vi "Read or Write Bookmark (XML file).vi"(1 "Read or write":enum16{"Read", "Write"}(ring)=enum."Write", 2 "Type":T1, 5 "PDF path file":path=path "C:/Users/JMS/Documents/PDF Report/Essais pdf/User Manual.pdf", 7 "XML File":path=path "C:/Users/JMS/Documents/PDF Report/Essais pdf/outline_actions31.xml", 11 "error in (no error)":errorcluster) -> (4 "GetBookmark":refnum<k24>, 6 "Bookmark?":bool, 8 "XML File duplicate":path=path "C:/Users/JMS/Documents/PDF Report/Essais pdf/outline_actions31.xml", 15 "error out":errorcluster)   [LabVIEW 2019, in "Exaprom PDF.lvlib"]
doc: "Version 1.1\nDeveloped by Jean-Marc Simard\nCopyright © 2012, Exaprom Inc.\nAll rights reserved.\nLicense: BSD\n\nWith iTextSharp 4.1.6 (http://itextsharp.sourceforge.net)\nunder Mozilla Public License Version 1.1\n(http://www.mozilla.org/MPL/MPL-1.1.html)"
uses:
  Controls/Text Controls/Unicode/Character type.ctl
  Controls/General Controls/Create, open or close.ctl
  Controls/Concatenate Controls/PDF file to concatenate.ctl
  C:/work/niobrara_lv/labview pdf writer fixing/DLL/itextsharp.dll
  DLL/itextsharp.dll
  Exaprom PDF.lvlib
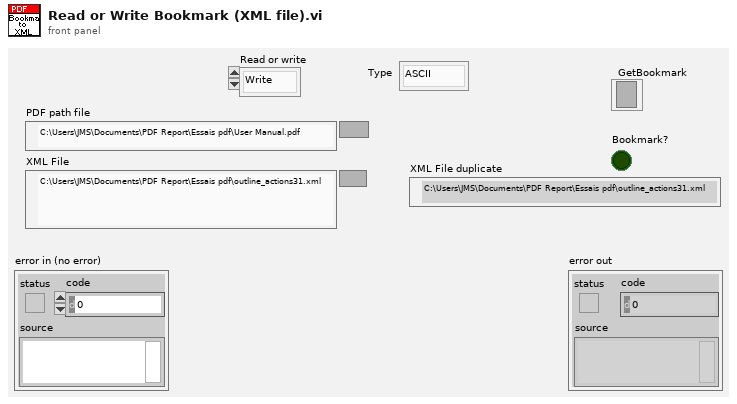
[diagram p1: front panel]
types:
  T1 = typedef "Exaprom PDF.lvlib/Character type.ctl" = enum16{"ASCII", "Unicode"}
  T2 = typedef "Exaprom PDF.lvlib/PDF file to concatenate.ctl" = cluster{"Path":path, "Pages":string, "Password":string}
  T3 = typedef "Exaprom PDF.lvlib/Create, open or close.ctl" = enum16{"Create", "Open", "Close"}
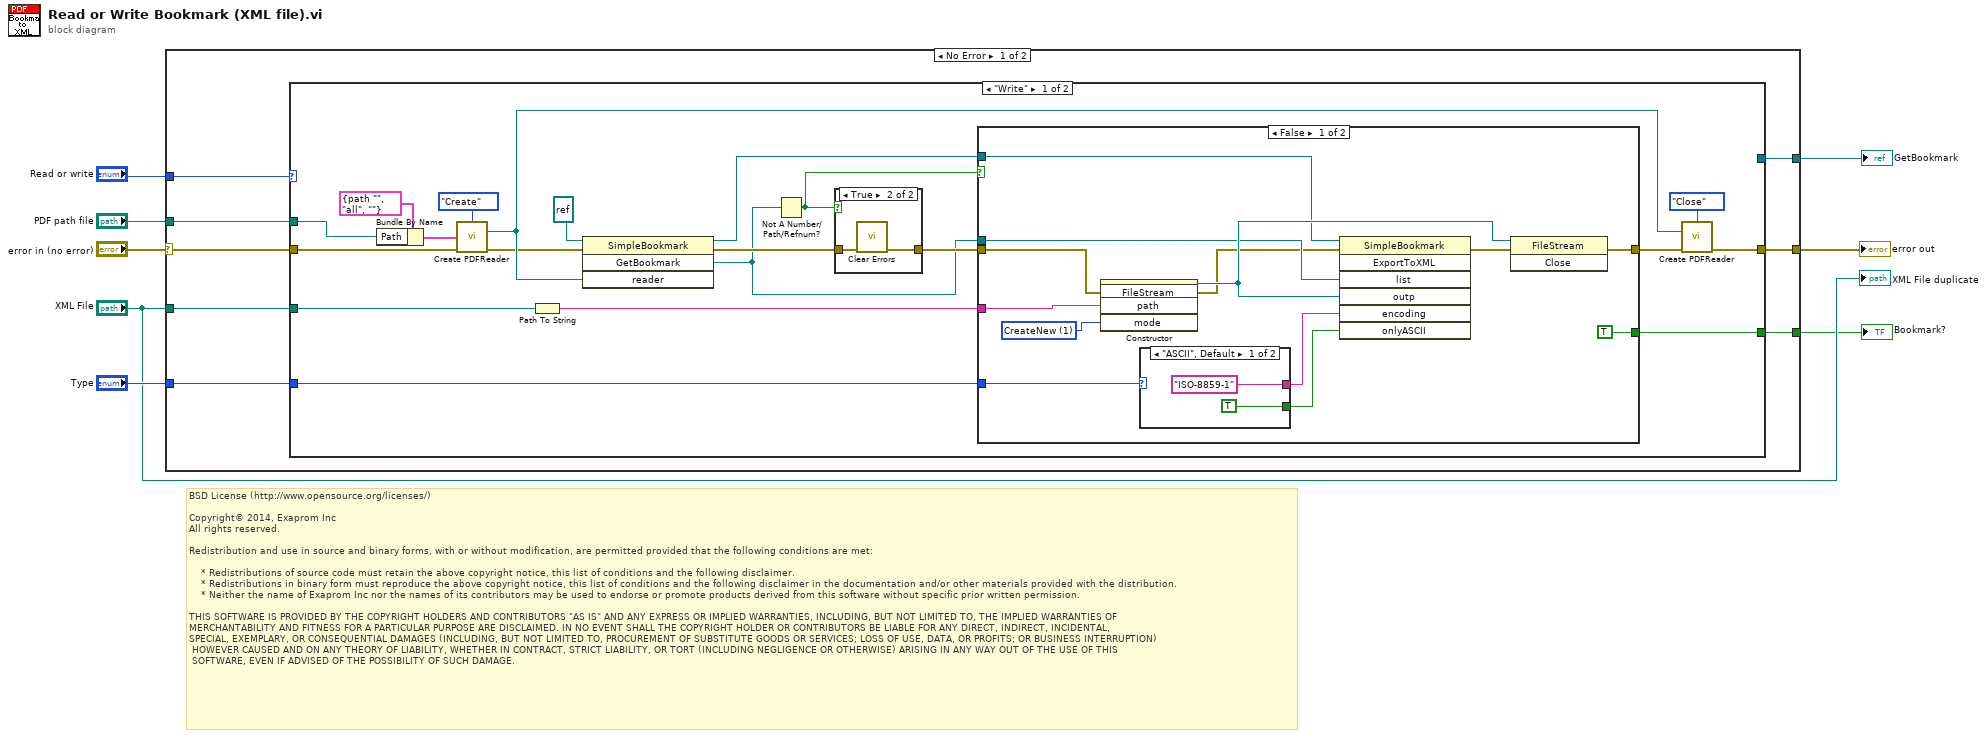
[diagram p0: block diagram]
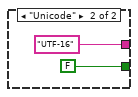
[diagram p3: hidden frame]
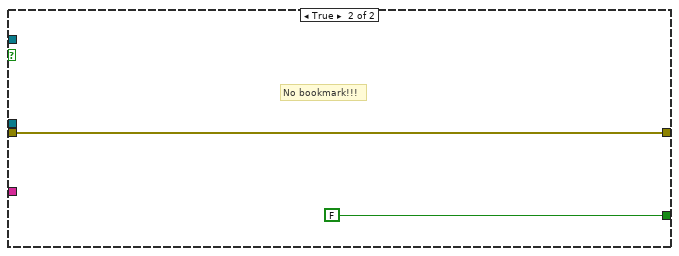
[diagram p4: hidden frame]
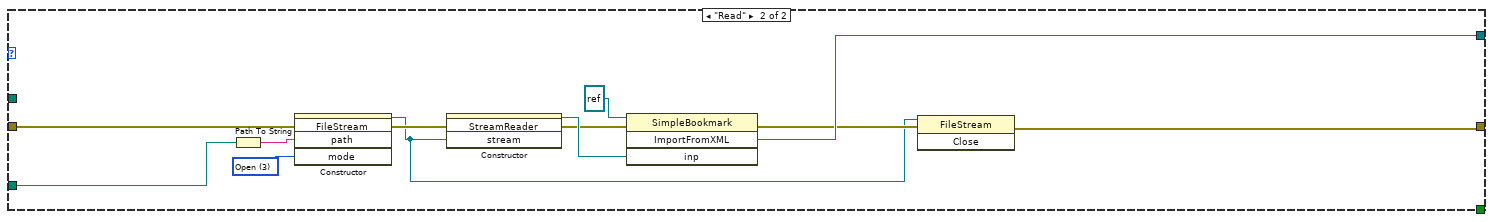
[diagram p5: hidden frame]
diagram:
  # "BSD License (http://www.opensource.org/licenses/)\n\nCopyright© 2014, Exaprom Inc\nAll rights reserved.\n\nRedistribution and use in source and binary forms, with or without modification, are permitted provided that the following conditions are met:\n\n    * Redistributions of source code must retain the above copyright notice, this list of conditions and the following disclaimer.\n    * Redistributions in binary form must reproduce the above copyright notice, this list of conditions and the following disclaimer in the documentation and/or other materials provided with the distribution.\n    * Neither the name of Exaprom Inc nor the names of its contributors may be used to endorse or promote products derived from this software without specific prior written permission.\n\nTHIS SOFTWARE IS PROVIDED BY THE COPYRIGHT HOLDERS AND CONTRIBUTORS \"AS IS\" AND ANY EXPRESS OR IMPLIED WARRANTIES, INCLUDING, BUT NOT LIMITED TO, THE IMPLIED WARRANTIES OF \nMERCHANTABILITY AND FITNESS FOR A PARTICULAR PURPOSE ARE DISCLAIMED. IN NO EVENT SHALL THE COPYRIGHT HOLDER OR CONTRIBUTORS BE LIABLE FOR ANY DIRECT, INDIRECT, INCIDENTAL,\nSPECIAL, EXEMPLARY, OR CONSEQUENTIAL DAMAGES (INCLUDING, BUT NOT LIMITED TO, PROCUREMENT OF SUBSTITUTE GOODS OR SERVICES; LOSS OF USE, DATA, OR PROFITS; OR BUSINESS INTERRUPTION)\n HOWEVER CAUSED AND ON ANY THEORY OF LIABILITY, WHETHER IN CONTRACT, STRICT LIABILITY, OR TORT (INCLUDING NEGLIGENCE OR OTHERWISE) ARISING IN ANY WAY OUT OF THE USE OF THIS\n SOFTWARE, EVEN IF ADVISED OF THE POSSIBILITY OF SUCH DAMAGE."
  n1 = case shown="No Error" "error in (no error)" {
    selector: "error in (no error)" -> [w14 w71]
    tunnel: [w13 w71] -> w8
    tunnel: "PDF path file" -> [w16 _]
    tunnel: "XML File" -> [w15 _]
    tunnel: "Type" -> [w12 _]
    tunnel: "Read or write" -> [w11 _]
    tunnel: [w10 _] -> w2
    tunnel: [w9 _] -> w1
    frame No Error {
      n2 = case shown="\"Write\"" w11 {
        tunnel: w16 -> [w30 _]
        tunnel: w15 -> [w29 w66]
        tunnel: w14 -> [w28 w67]
        tunnel: [w27 w60] -> w13
        tunnel: w12 -> [w26 _]
        tunnel: [_ w62] -> w10
        tunnel: [w22 _] -> w9
        frame "Write" {
          n3 = Bundle By Name(cluster=T2 {"Path"=path "", "Pages"="all", "Password"=""} ("File and pages"), "Path"=w30) -> (w31:T2)
          n4 = call "Create PDFReader.vi"("Action"=Create,_open_or_close."Create", "File and pages"=w31, "error in (no error)"=w28) -> ("PdfReader OUT"=w23:refnum<k24>, "error out"=w19:errorcluster)  [unwired: 9 in, 2 out]
          n5 = Path To String(path=w29) -> (string=w33:string)
          n6 = invoke class="SimpleBookmark" method="GetBookmark"(reference=refnum<k24> refnum ("new reference"), error in=w19, "reader"=w23) -> (reference out=w24:refnum<k24>, error out=w20:errorcluster, "GetBookmark"=w17:refnum<k24>)  [unwired: 1 in, 1 out]
          n7 = Not A Number/Path/Refnum?(number/path/refnum=w17) -> (NaN/Path/Refnum?=w18:bool)
          n8 = case shown="True" w18 {
            tunnel: [w37 w39] -> w21
            tunnel: w20 -> [w37 w38]
            frame False {
            }
            frame True {
              n9 = call <vilib>:"Clear Errors.vi"("error in (no error)"=w38) -> ("error out"=w39:errorcluster)  [unwired: 5 in, 1 out]
            }
          }
          n10 = case shown="False" w18 {
            tunnel: w33 -> [w50 _]
            tunnel: w26 -> [w48 _]
            tunnel: [w45 w58] -> w25
            tunnel: w24 -> [w44 _]
            tunnel: w17 -> [w43 _]
            tunnel: w21 -> [w42 w58]
            tunnel: [TRUE FALSE] -> w22
            frame False {
              w49 = 1 items=["CreateNew"=1, "Create"=2, "Open"=3, "OpenOrCreate"=4, "Truncate"=5, "Append"=6] ("mode")
              n11 = constructor class="FileStream" ("Constructor Node")(error in=w42, "path"=w50, "mode"=w49) -> (reference out=w47:refnum<k24>, error out=w41:errorcluster)  [unwired: 2 in, 3 out]
              n12 = case shown="\"ASCII\", Default" w48 {
                tunnel: ["ISO-8859-1" ("encoding") "UTF-16" ("encoding")] -> w52
                tunnel: [TRUE ("onlyASCII") FALSE ("onlyASCII")] -> w51
                frame "ASCII", Default {
                }
                frame "Unicode" {
                }
              }
              n13 = invoke class="SimpleBookmark" method="ExportToXML"(reference=w44, error in=w41, "list"=w43, "outp"=w47, "encoding"=w52, "onlyASCII"=w51) -> (error out=w46:errorcluster)  [unwired: 1 in, 6 out]
              n14 = invoke class="FileStream" method="Close"(reference=w47, error in=w46) -> (error out=w45:errorcluster)  [unwired: 1 in, 2 out]
            }
            frame True {
              # "No bookmark!!!"
            }
          }
          n15 = call "Create PDFReader.vi"("Action"=Create,_open_or_close."Close", "PdfReader IN"=w23, "error in (no error)"=w25) -> ("error out"=w27:errorcluster)  [unwired: 9 in, 3 out]
        }
        frame "Read" {
          w68 = 3 items=["CreateNew"=1, "Create"=2, "Open"=3, "OpenOrCreate"=4, "Truncate"=5, "Append"=6] ("mode")
          n16 = Path To String(path=w66) -> (string=w69:string)
          n17 = constructor class="FileStream" ("Constructor Node")(error in=w67, "path"=w69, "mode"=w68) -> (reference out=w59:refnum<k24>, error out=w64:errorcluster)  [unwired: 2 in, 3 out]
          n18 = constructor class="StreamReader" ("Constructor Node")(error in=w64, "stream"=w59) -> (reference out=w65:refnum<k24>, error out=w63:errorcluster)  [unwired: 2 in, 2 out]
          n19 = invoke class="SimpleBookmark" method="ImportFromXML"(reference=refnum<k24> refnum ("new reference"), error in=w63, "inp"=w65) -> (error out=w61:errorcluster, "ImportFromXML"=w62:refnum<k24>)  [unwired: 1 in, 2 out]
          n20 = invoke class="FileStream" method="Close"(reference=w59, error in=w61) -> (error out=w60:errorcluster)  [unwired: 1 in, 2 out]
        }
      }
    }
    frame Error {
    }
  }
  "error out" <- w8
  "GetBookmark" <- w2
  "Bookmark?" <- w1
  "XML File duplicate" <- "XML File"
